vi "Test UI Controls with Unicode.vi"() -> ()   [LabVIEW 2009]
uses:
  Tool_Unicode Update String.vi
panel:
  in  "Ring 2":u16(ring) caption="Selection" items=["Option A", "Option B", "Option C"]
  in  "Ring 3":i8(ring) caption="Selection" items=["Option A", "Option B", "Option C"]
  in  "Stop":bool
  out "Gauge":dbl(knob) scale=0.0..10.0
  in  "Boolean":bool caption="Switch"
  in  "Ring":u16(ring) caption="Selection" items=["Option A", "Option B", "Option C"]
  out "String":string="Menu" caption="ASCII Display"
  out "Table Control":string[][](table)=[["Option A"], ["Option B"], ["Option C"]] caption="Option A"
  in  "Language Selection":enum16{"English", "Japanese"}(ring)
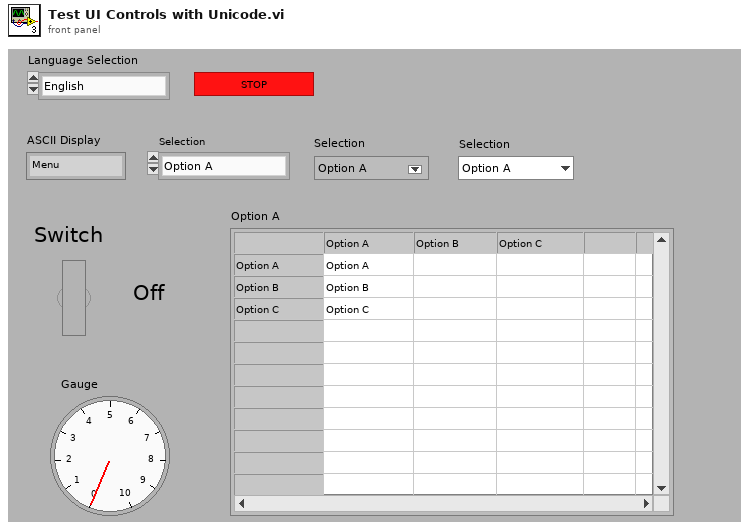
[diagram p1: front panel]
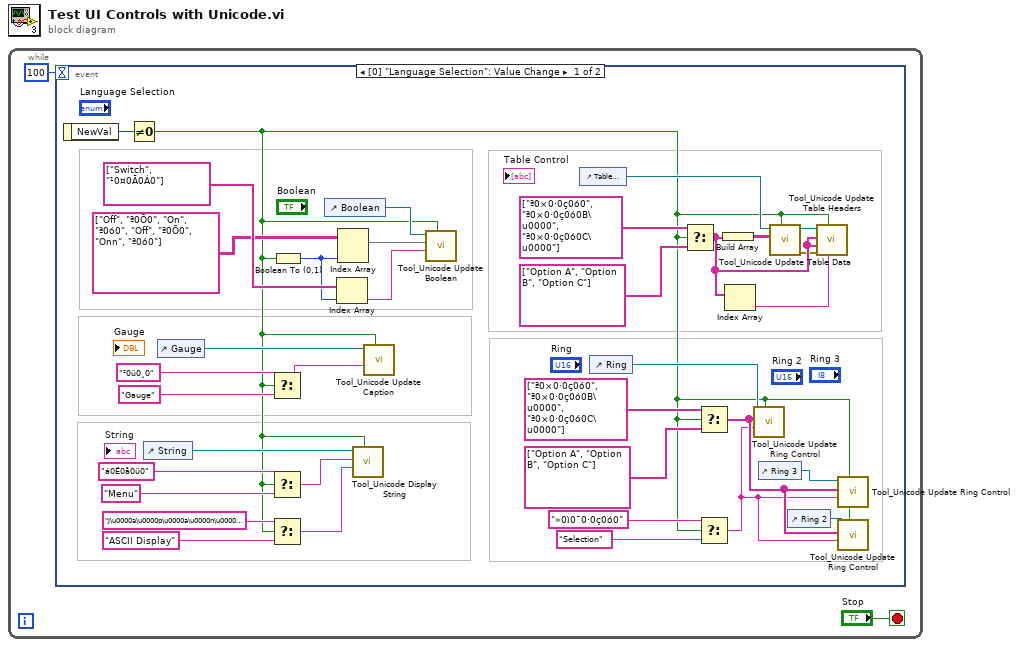
[diagram p0: block diagram]
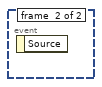
[diagram p2: hidden frame]
diagram:
  n1 = while {
    stop <- "Stop" stop-if-true
    n2 = event shown="[0] \"Language Selection\": Value Change" {
      selector: _ -> [_ _]
      dyn-events: _ -> [_ _]
      timeout: 100 -> [_ _]
      event #0 {
        n3 = event-data() -> ("NewVal"=w5:enum16{"English", "Japanese"})  [unwired: 1 in]
        n4 = Not Equal To 0?(x=w5) -> (x != 0?=w3:bool)
        n5 = control-ref of="String"() -> (w27:refnum<vi>)
        n6 = control-ref of="Gauge"() -> (w14:refnum<vi>)
        n7 = Select(t="²0ü0¸0" ("Caption"), s=w3, f="Gauge" ("Caption")) -> (s? t:f=w11:string)
        n8 = Select(t="á0Ë0å0ü0" ("Caption"), s=w3, f="Menu" ("Caption")) -> (s? t:f=w15:string)
        n9 = Select(t="J\u0000a\u0000p\u0000a\u0000n\u0000e\u0000s\u0000e\u0000 \u0000D\u0000i\u0000s\u0000p\u0000l\u0000a\u0000y\u0000" ("String"), s=w3, f="ASCII Display" ("Caption")) -> (s? t:f=w20:string)
        n10 = Boolean To (0,1)(Boolean=w3) -> (0, 1=w21:i16)
        n11 = control-ref of="Boolean"() -> (w26:refnum<vi>)
        n12 = Index Array(array=string[] ["Switch", "¹0¤0Ã0Á0"], index=w21) -> (element=w23:string)
        n13 = Index Array(array=string[][] [["Off", "ª0Õ0"], ["On", "ª0ó0"], ["Off", "ª0Õ0"], ["Onn", "ª0ó0"]], index (col)=w21) -> (element=w22:string[])  [unwired: 1 in]
        n14 = call "Tool_Unicode Display String.vi"("Interpret as Unicode (T)"=w3, "Caption"=w20, "String Value"=w15, "String Control Reference"=w27) -> ()  [unwired: 4 in, 2 out]
        n15 = call "Tool_Unicode Update Caption.vi"("Interpret as Unicode (T)"=w3, "Caption"=w11, "Control Reference"=w14) -> ()  [unwired: 5 in, 2 out]
        n16 = call "Tool_Unicode Update Boolean.vi"("Interpret as Unicode (T)"=w3, "Caption"=w23, "Boolean Texts [4]"=w22, "Boolean Reference"=w26) -> ()  [unwired: 4 in, 2 out]
        n17 = control-ref of="Table Control"() -> (w35:refnum<vi>)
        n18 = control-ref of="Ring"() -> (w30:refnum<vi>)
        n19 = Select(t=string[] ["ª0×0·0ç0ó0", "ª0×0·0ç0ó0B\u0000", "ª0×0·0ç0ó0C\u0000"], s=w3, f=string[] ["Option A", "Option B", "Option C"]) -> (s? t:f=w32:string[])
        n20 = Select(t=string[] ["ª0×0·0ç0ó0", "ª0×0·0ç0ó0B\u0000", "ª0×0·0ç0ó0C\u0000"], s=w3, f=string[] ["Option A", "Option B", "Option C"]) -> (s? t:f=w7:string[])
        n21 = Select(t="»0ì0¯0·0ç0ó0" ("String"), s=w3, f="Selection" ("Caption")) -> (s? t:f=w6:string)
        n22 = Build Array(w32) -> (w36:string[][])
        n23 = Index Array(array=w32) -> (element=w33:string)  [unwired: 1 in]
        n24 = call "Tool_Unicode Update Ring Control.vi"("Interpret as Unicode (T)"=w3, "Caption"=w6, "Strings"=w7, "Ring Control Ref"=w30) -> ()  [unwired: 5 in, 1 out]
        n25 = control-ref of="Ring 3"() -> (w8:refnum<vi>)
        n26 = call "Tool_Unicode Update Table Data.vi"("Interpret as Unicode (T)"=w3, "Data[]"=w36, "Table Ref"=w35) -> ("error out"=w31:errorcluster, "Table Ref"=w34:refnum<vi>)  [unwired: 5 in]
        n27 = control-ref of="Ring 2"() -> (w4:refnum<vi>)
        n28 = call "Tool_Unicode Update Table Headers.vi"("Caption"=w33, "Interpret as Unicode (T)"=w3, "error in (no error)"=w31, "Row Headers[]"=w32, "Column Headers[]"=w32, "Table Ref"=w34) -> ()  [unwired: 4 in, 2 out]
        n29 = call "Tool_Unicode Update Ring Control.vi"("Interpret as Unicode (T)"=w3, "Caption"=w6, "Strings"=w7, "Ring Control Ref"=w8) -> ()  [unwired: 5 in, 1 out]
        n30 = call "Tool_Unicode Update Ring Control.vi"("Interpret as Unicode (T)"=w3, "Caption"=w6, "Strings"=w7, "Ring Control Ref"=w4) -> ()  [unwired: 5 in, 1 out]
      }
      event #1 {
        n31 = event-data() -> ()  [unwired: 1 in, 1 out]
      }
    }
  }
